vi "Trajectory_Execution_Begin.vi"   [LabVIEW 2019]
uses:
  Trajectory_Execution_Globals.vi
types:
  T1 = typedef "Trajectory_Library.lvlib/TRAJECTORY.ctl" = cluster{"TotalTImeSecs":dbl, "States":T2[]}
  T2 = typedef "Trajectory_Library.lvlib/TRAJ_STATE.ctl" = cluster{"TimeSeconds":dbl, "Velocity":dbl, "Acceleration":dbl, "POSE":T3, "Curvature":dbl}
  T3 = typedef "Trajectory_Library.lvlib/POSE2D.ctl" = cluster{"TRANSLATION":T4, "ROTATION":T5}
  T4 = typedef "Trajectory_Library.lvlib/TRANSLATION2D.ctl" = cluster{"X":dbl, "Y":dbl}
  T5 = typedef "Trajectory_Library.lvlib/ROTATION2D.ctl" = cluster{"VALUE":dbl, "COS":dbl, "SIN":dbl}
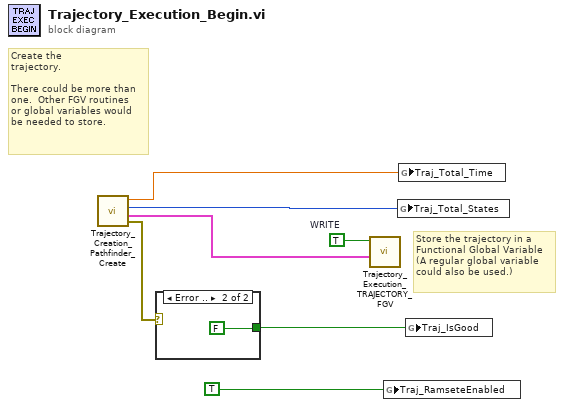
[diagram p0: block diagram]
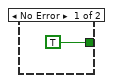
[diagram p2: hidden frame]
diagram:
  w2 = TRUE  # WRITE
  # "Store the trajectory in a \nFunctional Global Variable\n(A regular global variable\ncould also be used.)"
  # "Create the\ntrajectory.\n\nThere could be more than\none.  Other FGV routines\nor global variables would\nbe needed to store."
  n1 = call "Trajectory_Creation_Pathfinder_Create.vi"() -> ("Path calculation error"=w7:errorcluster, "Relative Trajectory"=w1:T1, "Trajectory Items"=w5:i32, "TotalTImeSecs"=w6:dbl)  [unwired: 8 in]
  n2 = case shown="Error .." w7 {
    tunnel: [TRUE FALSE] -> w4
    frame No Error {
    }
    frame Error {
    }
  }
  n3 = call "Trajectory_Execution_TRAJECTORY_FGV.vi"("inTRAJECTORY"=w1, "WRITE"=w2) -> ()  [unwired: 9 in, 1 out]
  n4 = global write "Trajectory_Execution_Globals.vi" "Traj_RamseteEnabled"(TRUE) -> ()
  n5 = global write "Trajectory_Execution_Globals.vi" "Traj_Total_States"(w5) -> ()
  n6 = global write "Trajectory_Execution_Globals.vi" "Traj_Total_Time"(w6) -> ()
  n7 = global write "Trajectory_Execution_Globals.vi" "Traj_IsGood"(w4) -> ()
